vi "_Construct Error Cluster.vi"(4 "error in":errorcluster, 5 "reason":string, 6 "CallingChain? (T)":bool=TRUE, 7 "errorCode":i32=8000) -> (0 "error out":errorcluster)   [LabVIEW 2015]
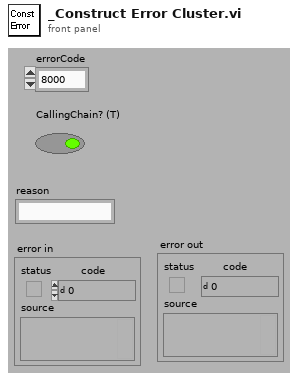
[diagram p1: front panel]
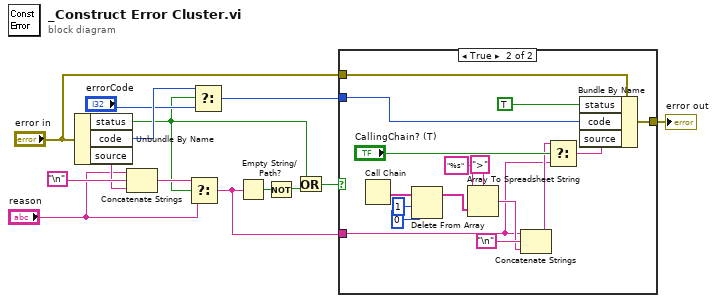
[diagram p0: block diagram]
diagram:
  n1 = Unbundle By Name("error in") -> ("status"=w8:bool, "code"=w14:i32, "source"=w2:string)
  n2 = Concatenate Strings("reason", "\n", w2) -> (w12:string)
  n3 = Select(t=w12, s=w8, f="reason") -> (s? t:f=w4:string)
  n4 = Select(t=w14, s=w8, f="errorCode") -> (s? t:f=w5:i32)
  n5 = Empty String/Path?(string/path=w4) -> (empty?=w10:bool)
  n6 = Not(x=w10) -> (.not. x?=w9:bool)
  n7 = Or(x=w8, y=w9) -> (x .or. y?=w7:bool)
  n8 = case shown="True" w7 {
    tunnel: [w15 w29] -> w3
    tunnel: "error in" -> [w15 w28]
    tunnel: w4 -> [_ w16]
    tunnel: w5 -> [_ w22]
    frame False {
      # "Empty string means no error"
    }
    frame True {
      n9 = Call Chain() -> (call chain=w26:string[])
      n10 = Delete From Array(array=w26, length=1, index=0) -> (array with subset deleted=w23:string[])  [unwired: 1 out]
      n11 = Array To Spreadsheet String(delimiter (Tab)=">", array=w23, 3:"%s" ("format string")) -> (spreadsheet string=w21:string)
      n12 = Concatenate Strings(w16, "\n", w21) -> (w18:string)
      n13 = Select(t=w18, s="CallingChain? (T)", f=w16) -> (s? t:f=w17:string)
      n14 = Bundle By Name(cluster=w28, "status"=TRUE, "code"=w22, "source"=w17) -> (w29:errorcluster)
    }
  }
  "error out" <- w3
